vi "LoadJSON.vi"() -> (0 "error out":errorcluster, 3 "JSON Tree out (JSON Array)":variant)   [LabVIEW 2018]
uses:
  Global Variables.vi
  <vilib>/LVH/i3 JSON/i3-json.lvlib
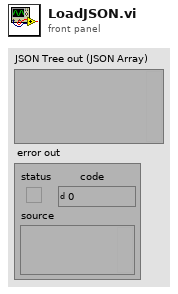
[diagram p1: front panel]
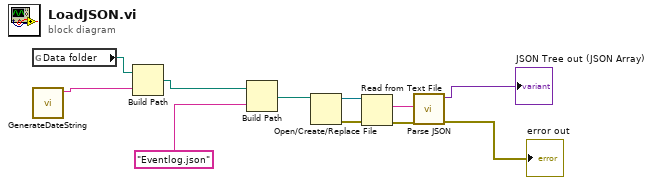
[diagram p0: block diagram]
diagram:
  n1 = global read "Global Variables.vi" "Data folder"() -> (w10:path)
  n2 = call "GenerateDateString.vi"() -> ("String"=w11:string)  [unwired: 11 in]
  n3 = Build Path(base path=w10, name or relative path=w11) -> (appended path=w9:path)
  n4 = Build Path(base path=w9, name or relative path="Eventlog.json" ("string")) -> (appended path=w7:path)
  n5 = Open/Create/Replace File(file path (use dialog)=w7) -> (refnum out=w6:refnum<file>, error out=w3:errorcluster)  [unwired: 5 in, 1 out]
  n6 = Read from Text File(file (use dialog)=w6, error in=w3) -> (text=w4:string, error out=w5:errorcluster)  [unwired: 2 in, 2 out]
  n7 = call <vilib>:"Parse JSON.vi"("error in (no error)"=w5, "JSON String"=w4) -> ("error out"=→"error out":errorcluster, "JSON Tree"=→"JSON Tree out (JSON Array)":variant)  [unwired: 6 in, 2 out]
